vi "Create Process.vi"(8 "error in (no error)":errorcluster, 11 "process name":string) -> (0 "error out":errorcluster, 3 "dup process name":string)   [LabVIEW 2018, in "Dynamic Shared Variables.lvlib"]
uses:
  Dynamic Shared Variables.lvlib
  <vilib>/lvdsc/NI_DSC.lvlib
panel:
  out "Database path":path
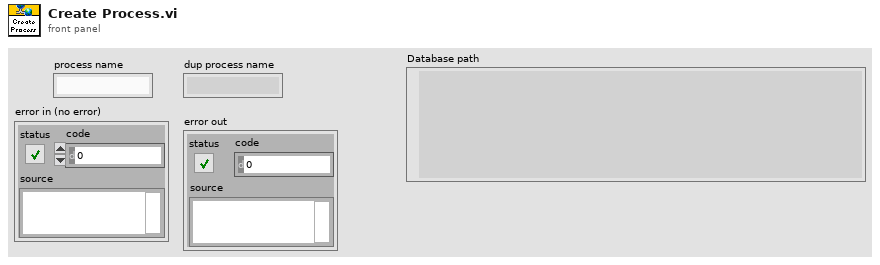
[diagram p1: front panel]
types:
  T1 = cluster{"machine":string, "name":string, "path":path}
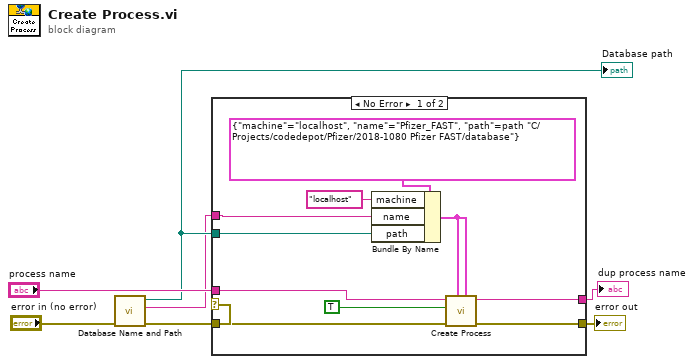
[diagram p0: block diagram]
diagram:
  n1 = call "Database Name and Path.vi"("error in (no error)"="error in (no error)") -> ("error out"=w1:errorcluster, "database name"=w3:string, "databse path"=w4:path)  [unwired: 8 in]
  "Database path" <- w4
  n2 = case shown="No Error" w1 {
    tunnel: [w17 w18] -> w7
    tunnel: [w16 w19] -> w6
    tunnel: "process name" -> [w11 w18]
    tunnel: w1 -> [w14 w19]
    tunnel: w4 -> [w10 _]
    tunnel: w3 -> [w8 _]
    frame No Error {
      n3 = Bundle By Name(cluster=T1 {"machine"="localhost", "name"="Pfizer_FAST", "path"=path "C:/Projects/codedepot/Pfizer/2018-1080 Pfizer FAST/database"} ("data database"), "machine"="localhost", "name"=w8, "path"=w10) -> (w12:T1)
      n4 = call <vilib>:"Create Process.vi"("alarm database"=w12, "data database"=w12, "error in (no error)"=w14, "run?"=TRUE, "process name"=w11) -> ("error out"=w16:errorcluster, "process name out"=w17:string)  [unwired: 5 in]
    }
    frame Error {
    }
  }
  "dup process name" <- w7
  "error out" <- w6
